vi "writetofile.vi"(0 "reference":refnum<vi>) -> ()   [LabVIEW 2019]
uses:
  Global 1.vi
  <vilib>/Utility/file.llb/Write Delimited Spreadsheet (string).vi
panel:
  out "path":path
  in  "Numeric":dbl
  out "error out":errorcluster
  out "Boolean":bool
  out "He3 Pressure\n(Torr)":dbl
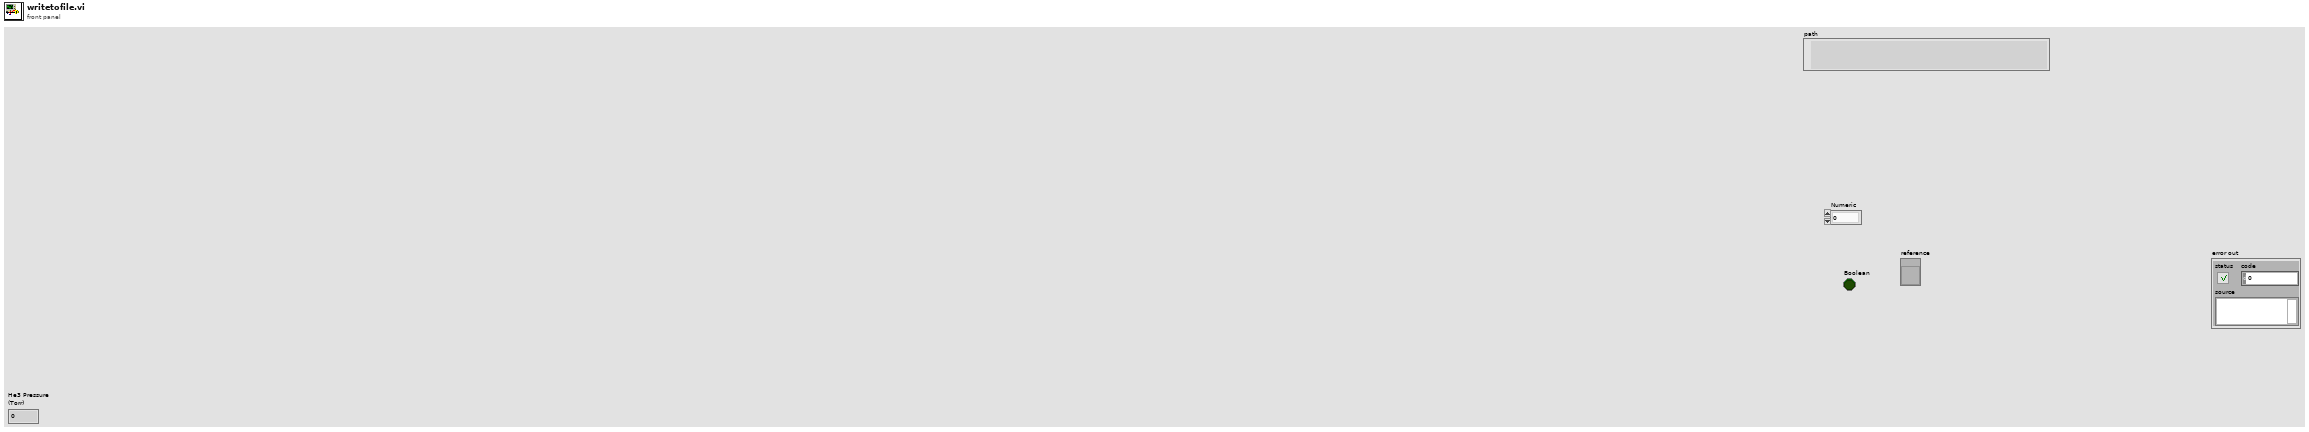
[diagram p1: front panel]
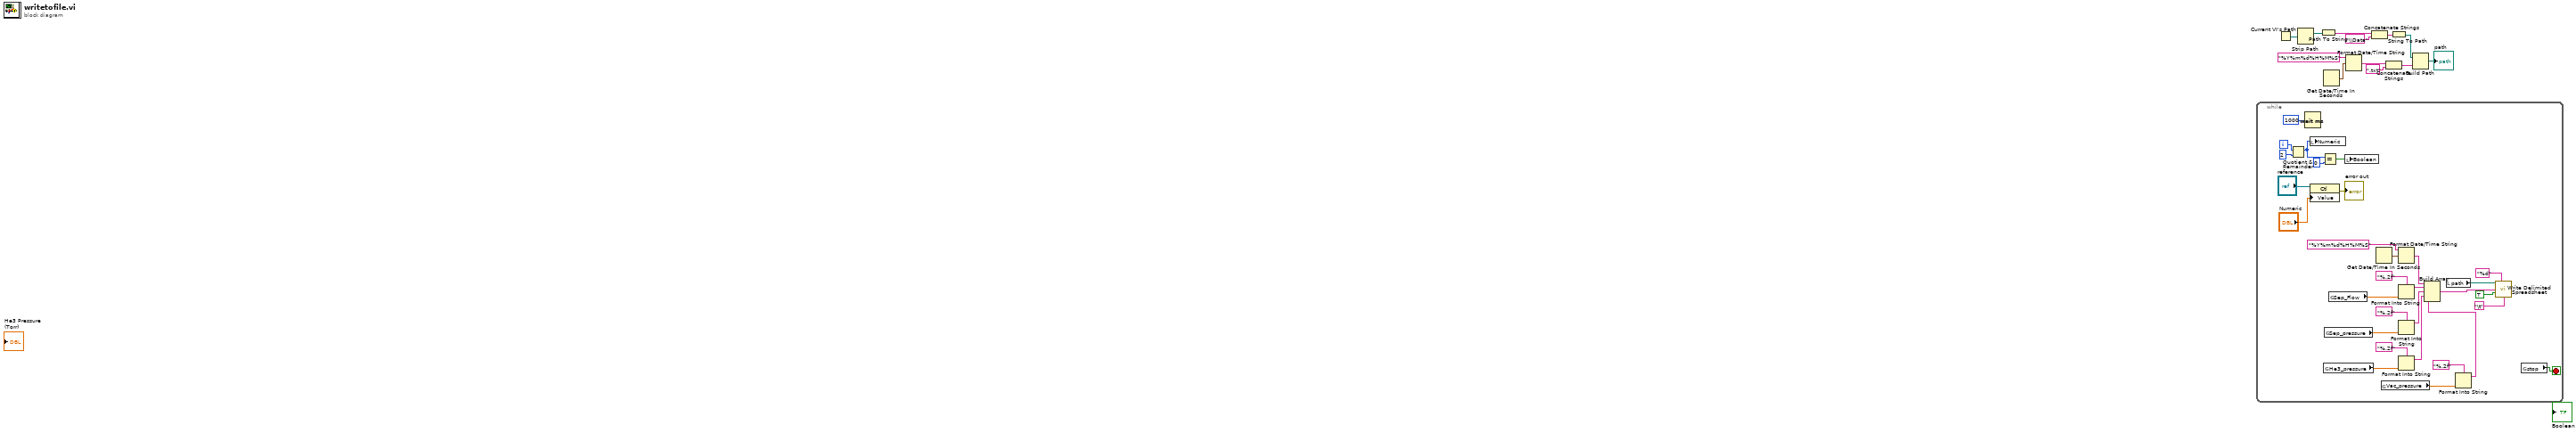
[diagram p0: block diagram]
diagram:
  n1 = while {
    i -> [w27]
    stop <- w29 stop-if-true
    n2 = Quotient & Remainder(x=w27, y=2) -> (x-y*floor(x/y)=w23:i32)  [unwired: 1 out]
    n3 = Wait (ms)(milliseconds to wait=u32 1000) -> ()  [unwired: 1 out]
    n4 = local write "Numeric"(w23) -> ()
    n5 = property class="Ctl"(reference="reference", "Value"="Numeric") -> (error out=→"error out":errorcluster)  [unwired: 1 in, 1 out]
    n6 = Equal?(x=w23, y=0) -> (x = y?=w24:bool)
    n7 = global read "Global 1.vi" "He3_pressure"() -> (w31:dbl)
    n8 = global read "Global 1.vi" "Sep_pressure"() -> (w32:dbl)
    n9 = global read "Global 1.vi" "Sep_Flow"() -> (w30:dbl)
    n10 = local write "Boolean"(w24) -> ()
    n11 = Get Date/Time In Seconds() -> (seconds since 1Jan1904=w18:timestamp)
    n12 = global read "Global 1.vi" "Vac_pressure"() -> (w14:dbl)
    n13 = Format Date/Time String(time format string (%c)="%Y%m%d%H%M%S", seconds (now)=w18) -> (date/time string=w17:string)  [unwired: 1 in]
    n14 = Format Into String(format string="%.2f", w30) -> (resulting string=w37:string)  [unwired: 2 in, 1 out]
    n15 = Format Into String(format string="%.2f", w32) -> (resulting string=w35:string)  [unwired: 2 in, 1 out]
    n16 = Format Into String(format string="%.2f", w31) -> (resulting string=w33:string)  [unwired: 2 in, 1 out]
    n17 = local read "path"() -> (w16:path)
    n18 = Format Into String(format string="%.2f", w14) -> (resulting string=w13:string)  [unwired: 2 in, 1 out]
    n19 = Build Array(w17, w37, w35, w33, w13) -> (w42:string[])
    n20 = call-poly <vilib>:"Write Delimited Spreadsheet.vi"("file path (dialog if empty)"=w16, "format (%s)"="%d" ("format (%.3f)"), "1D data"=w42, "append to file? (new file:F)"=TRUE, "delimiter (\\t)"="\t" ("delimiter (\\t)")) -> ()  [unwired: 9 in, 2 out]
    n21 = global read "Global 1.vi" "stop"() -> (w29:bool)
  }
  n22 = Current VI's Path() -> (path=w6:path)
  n23 = Strip Path(path=w6) -> (stripped path=w4:path)  [unwired: 1 out]
  n24 = Path To String(path=w4) -> (string=w3:string)
  n25 = Get Date/Time In Seconds() -> (seconds since 1Jan1904=w11:timestamp)
  n26 = Format Date/Time String(time format string (%c)="%Y%m%d%H%M%S", seconds (now)=w11) -> (date/time string=w8:string)  [unwired: 1 in]
  n27 = Concatenate Strings(w3, "\\Data" ("string")) -> (w2:string)
  n28 = Concatenate Strings(w8, ".txt" ("string")) -> (w9:string)
  n29 = String To Path(string=w2) -> (path=w1:path)
  n30 = Build Path(base path=w1, name or relative path=w9) -> (appended path=→"path":path)
